vi "Rendezvous_1.vi"() -> ()   [LabVIEW 2019]
uses:
  <vilib>/Platform/TimedLoop/XDataNode/timing_clust.ctl
  <vilib>/Platform/TimedLoop/XDataNode/nitl_modes.ctl
  <vilib>/Platform/TimedLoop/XDataNode/wakeup.ctl
  <vilib>/Platform/TimedLoop/scheduler/LVUserAPI/_suppVIs/Create_1kHz_TSource.vi
  <vilib>/platform/TimedLoop/XDataNode/XDataNode.xnode
  <vilib>/Platform/TimedLoop/XDataNode/XDNodeRunTimeDep.lvlib
panel:
  out "Dioda":bool
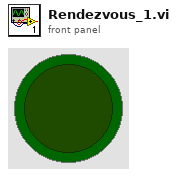
[diagram p1: front panel]
types:
  T1 = typedef "XDNodeRunTimeDep.lvlib/timing_clust.ctl" = cluster{"Expected End [f-1]":u64, "Actual End [f-1]":u64, "Finished Late? [f-1]":bool, "Expected End [i-1]":u64, "Actual End [i-1]":u64, "Finished Late? [i-1]":bool, "Expected Start [i]":u64, "Actual Start [i]":u64, "Expected Start [f]":u64, "Actual Start [f]":u64, "Source Name":string, "Structure Name":string, "Period":i64, "Deadline":i64, "Offset":i64, "Start":i64, "Priority":i32, "Timeout":i32, "Mode":T2, "Wakeup Reason":T3, "Error":errorcluster, "Source Type":string, "Secondary Source Type":string, "Global End Time":u64, "Global Start Time":u64, "Frame Duration":u64, "Iteration Duration":u64, "Assigned CPU":i32, "I/O Scan Engine Mode":u32}
  T2 = typedef "XDNodeRunTimeDep.lvlib/nitl_modes.ctl" = enum32{"No Change", "Process missed periods, maintain original phase", "Discard missed periods, maintain original phase", "Process missed periods, ignore original phase", "Discard missed periods, ignore original phase"}
  T3 = typedef "XDNodeRunTimeDep.lvlib/wakeup.ctl" = enum32{"Normal", "Aborted", "Asynchronous wakeup", "Timing source error", "Timed loop error", "Timeout"}
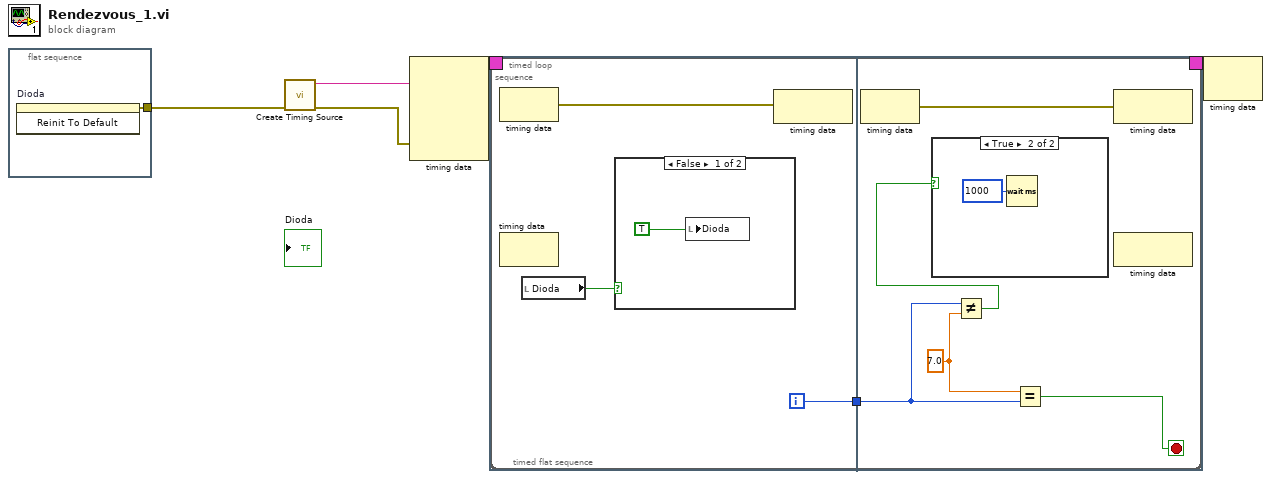
[diagram p0: block diagram]
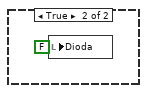
[diagram p2: hidden frame]
diagram:
  n1 = flat-sequence {
    tunnel: [w6] -> w1
    frame #0 {
      n2 = invoke on="Dioda" class="Bool (strict)" method="Reinit To Default"() -> (error out=w6:errorcluster)  [unwired: 3 in, 2 out]
    }
  }
  n3 = call-poly <vilib>:"Create Timing Source.vi"("error in (no error)"=w1) -> ("error out"=w2:errorcluster, "name (out)"=w3:string)  [unwired: 9 in]
  n4 = node-c288(w3, w2) -> (w5:T1)  [unwired: 3 in]
  n5 = timed-loop {
    timing: w5 -> [_]
    timing-out: [_] -> w4
    i -> [w8]
    stop <- w21 stop-if-true
    n6 = timed-sequence {
      timing: _ -> [_]
      timing-out: _ -> [_]
      n7 = timed-flat-sequence {
        tunnel: [w8] -> w7
        tunnel: w7 -> [w19]
        frame #0 {
          n8 = node-c288() -> (w10:errorcluster)  [unwired: 1 in]
          n9 = local read "Dioda"() -> (w9:bool)
          n10 = case shown="False" w9 {
            frame False {
              n11 = local write "Dioda"(TRUE ("LED")) -> ()
            }
            frame True {
              n12 = local write "Dioda"(FALSE ("LED")) -> ()
            }
          }
          n13 = node-c288(w10) -> ()  [unwired: 1 out]
        }
        frame #1 {
          w20 = 7.0 ("x")
          n14 = node-c288() -> (w22:errorcluster)  [unwired: 1 in]
          n15 = Not Equal?(x=w19, y=w20) -> (x != y?=w18:bool)
          n16 = case shown="True" w18 {
            frame False {
            }
            frame True {
              n17 = Wait (ms)(milliseconds to wait=u32 1000) -> ()  [unwired: 1 out]
            }
          }
          n18 = Equal?(x=w20, y=w19) -> (x = y?=w21:bool)
          n19 = node-c288(w22) -> ()  [unwired: 1 out]
        }
      }
    }
    n20 = node-c288() -> ()  [unwired: 1 in, 1 out]
    n21 = node-c288() -> ()  [unwired: 1 in, 1 out]
  }
  n22 = node-c288(w4) -> ()  [unwired: 1 out]
